vi "Read Data-String.vi"(6 "timeout ms":i32=5000, 8 "error in":errorcluster, 11 "NetStream in":refnum<class "NetStream.lvclass">) -> (0 "error out":errorcluster, 1 "Received bytes":i32, 2 "data out":string, 3 "NetStream out":refnum<class "NetStream.lvclass">)   [LabVIEW 2014, in "hse-network.lvlib" / "NetStream.lvclass"]
uses:
  NetStream.lvclass
  NetStream.lvclass/NetStream.ctl
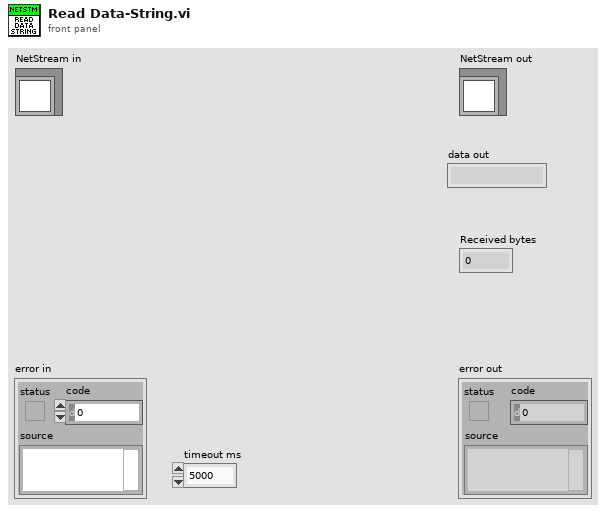
[diagram p1: front panel]
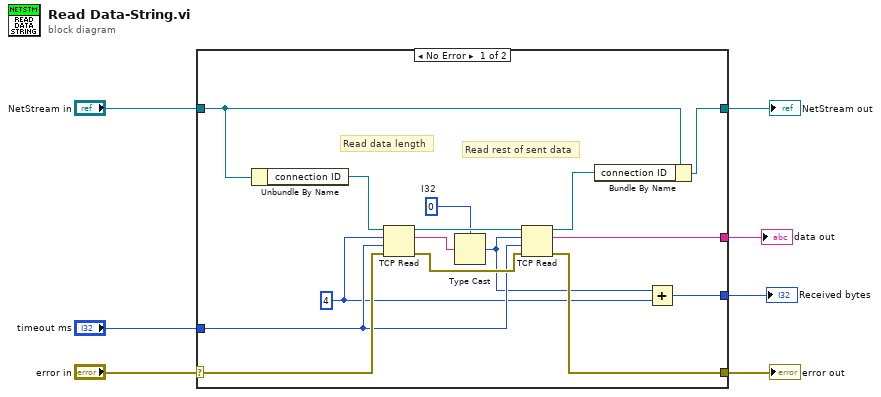
[diagram p0: block diagram]
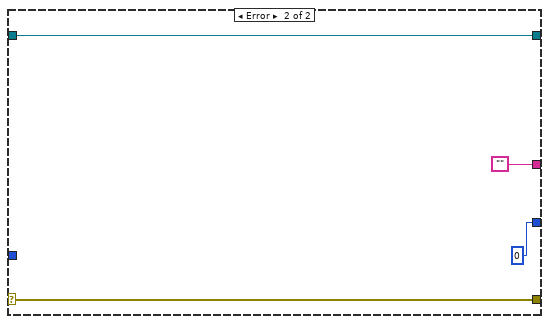
[diagram p2: hidden frame]
diagram:
  n1 = case shown="No Error" "error in" {
    selector: "error in" -> [w20 w26]
    tunnel: [w16 w26] -> w6
    tunnel: [w13 w25] -> w4
    tunnel: "NetStream in" -> [w14 w25]
    tunnel: "timeout ms" -> [w11 _]
    tunnel: [w15 ""] -> w2
    tunnel: [w10 0 ("timeout ms")] -> w1
    frame No Error {
      w18 = 0  # I32
      w9 = 4 ("bytes to read")
      # "Read rest of sent data"
      # "Read data length"
      n2 = Unbundle By Name(w14) -> ("connection ID"=w21:refnum<k5>)
      n3 = TCP Read(connection ID=w21, bytes to read=w9, error in (no error)=w20, 9:w11) -> (connection ID out=w19:refnum<k5>, data out=w17:string, error out=w22:errorcluster)  [unwired: 1 in]
      n4 = Type Cast(type=w18, x=w17) -> (*(type *) &x=w8:i32)
      n5 = TCP Read(connection ID=w19, bytes to read=w8, error in (no error)=w22, 9:w11) -> (connection ID out=w12:refnum<k5>, data out=w15:string, error out=w16:errorcluster)  [unwired: 1 in]
      n6 = Bundle By Name(cluster=w14, "connection ID"=w12) -> (w13:refnum<class "NetStream.lvclass">)
      n7 = Add(x=w8, y=w9) -> (x+y=w10:i32)
    }
    frame Error {
    }
  }
  "error out" <- w6
  "NetStream out" <- w4
  "data out" <- w2
  "Received bytes" <- w1
